vi "Secure WebSocket Client Test with dotNET - Read Timeout.vi"() -> ()   [LabVIEW 2013]
uses:
  dotNET SSL Socket/dotNET WebSocket/Client/SSL Client Options.ctl
  dotNET SSL Socket/dotNET SSL Socket/PFX Certificate.ctl
  dotNET SSL Socket/dotNET WebSocket/Client/dotNET WebSocket Client.lvclass
  <vilib>/MediaMongrels Ltd/WebSockets/WebSockets/WebSocket/WebSocket.lvclass/WebSocket.ctl
  <vilib>/MediaMongrels Ltd/WebSockets/WebSockets/WebSocket/Read Return Headers.vi
  <vilib>/MediaMongrels Ltd/WebSockets/WebSockets/WebSocket Client/WebSocket Client.lvclass
  dotNET SSL Socket/dotNET SSL Client/dotNET SSL Client Socket.lvclass
  dotNET SSL Socket/dotNET TCP Socket/dotNET TCP Socket.lvclass
  dotNET SSL Socket/dotNET SSL Socket/dotNET SSL Socket.lvclass
  NI OpenSSL Socket/SSL_Lib/SSL-Lib/SSL-Lib.lvclass
panel:
  out "x-y":u32
  out "error out 3":errorcluster
  out "Data 3":string
  out "error out 2":errorcluster
  out "error out":errorcluster
  out "Data":string
  out "Return Headers":variant
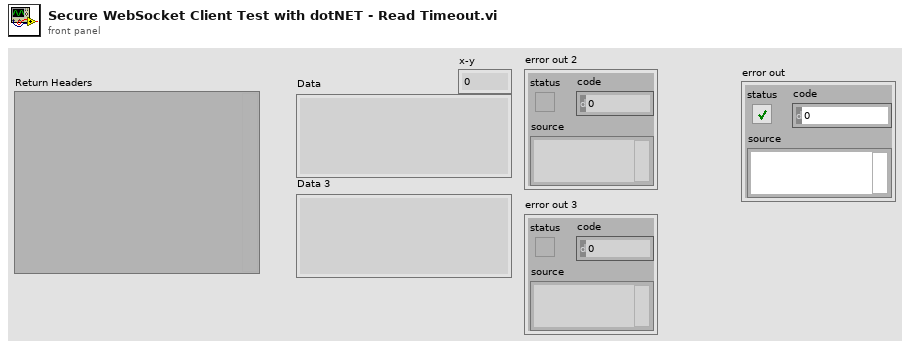
[diagram p1: front panel]
types:
  T1 = typedef "dotNET WebSocket.lvlib/dotNET WebSocket Client.lvclass/SSL Client Options.ctl" = cluster{"Check Revocation":bool, "SSL Protocols":i32[], "Client Certs":T2[]}
  T2 = typedef "dotNET SSL Socket.lvlib/dotNET SSL Socket.lvclass/PFX Certificate.ctl" = cluster{"PFX Certificate":path, "PFX Password":string}
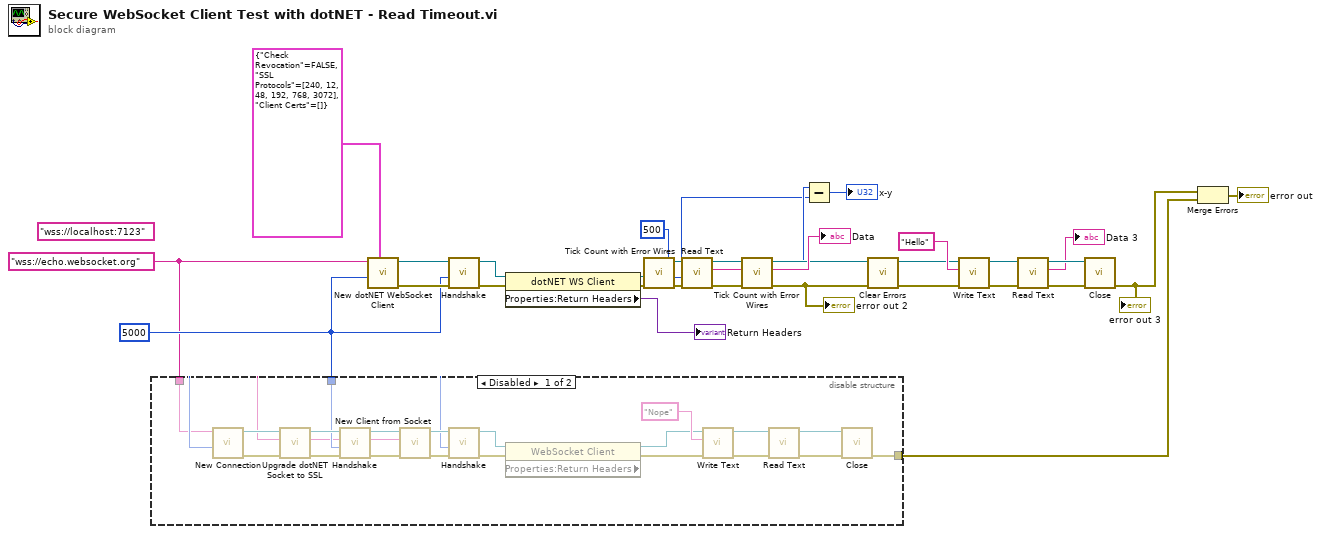
[diagram p0: block diagram]
diagram:
  (unwired) "wss://localhost:7123" ("WebSocket URL")
  w21 = 5000 ("Timeout (5000ms)")
  w19 = "wss://echo.websocket.org" ("WebSocket URL")
  n1 = disable-structure shown="Disabled" {
    disable-tunnel: [w51 _] -> w25
    disable-tunnel: w21 -> [w31 _]
    disable-tunnel: w19 -> [w30 _]
    frame Disabled {
      n2 = call "New Connection.vi"("Timeout (5000ms)"=w31, "Hostname / URL"=w30) -> ("error out"=w32:errorcluster, "dotNET TCP Socket out"=w36:refnum<class "dotNET TCP Socket.lvclass">)  [unwired: 8 in]
      n3 = call "Upgrade dotNET Socket to SSL.vi"("error in (no error)"=w32, "Hostname / URL"=w30, "dotNET TCP Socket in"=w36) -> ("error out"=w33:errorcluster, "dotNET SSL Client Socket out"=w37:refnum<class "dotNET SSL Client Socket.lvclass">)  [unwired: 7 in]
      n4 = call-dynamic "Handshake.vi"("error in (no error)"=w33, "Timeout (5000ms)"=w31, "dotNET SSL Client Socket in"=w37) -> ("error out"=w34:errorcluster, "dotNET SSL Client Socket out"=w35:refnum<class "dotNET SSL Client Socket.lvclass">)  [unwired: 7 in]
      n5 = call <vilib>:"New Client from Socket.vi"("error in (no error)"=w34, "WebSocket URL"=w30, "Socket in"=w35) -> ("error out"=w38:errorcluster, "WebSocket Client out"=w39:refnum<class "WebSocket Client.lvclass">)  [unwired: 7 in]
      n6 = call-dynamic "Handshake.vi"("error in (no error)"=w38, "timeout ms (5000)"=w31, "WebSocket Client in"=w39) -> ("error out"=w40:errorcluster, "WebSocket Client out"=w41:refnum<class "WebSocket Client.lvclass">)  [unwired: 7 in]
      n7 = property class="WebSocket Client"(reference=w41, error in=w40) -> (reference out=w44:refnum<class "WebSocket Client.lvclass">, error out=w43:errorcluster, "Properties:Return Headers"=w42:variant)
      n8 = call-dynamic "Write Text.vi"("error in (no error)"=w43, "String Data"="Nope", "WebSocket in"=w44) -> ("error out"=w46:errorcluster, "WebSocket out"=w47:refnum<class "WebSocket Client.lvclass">)  [unwired: 7 in]
      n9 = call-dynamic "Read Text.vi"("error in (no error)"=w46, "WebSocket in"=w47) -> ("error out"=w49:errorcluster, "Data"=w48:string, "WebSocket out"=w50:refnum<class "WebSocket Client.lvclass">)  [unwired: 7 in]
      n10 = call-dynamic "Close.vi"("error in (no error)"=w49, "WebSocket in"=w50) -> ("error out"=w51:errorcluster)  [unwired: 9 in]
    }
    frame Enabled {
    }
  }
  n11 = call "New dotNET WebSocket Client.vi"("Client SSL Options (wss://)"=T1 {"Check Revocation"=FALSE, "SSL Protocols"=[240, 12, 48, 192, 768, 3072], "Client Certs"=[]} ("SSL Options (for wss://)"), "Timeout (5000ms)"=w21, "WebSocket URL"=w19) -> ("error out"=w23:errorcluster, "dotNET WS Client out"=w22:refnum<class "dotNET WebSocket Client.lvclass">)  [unwired: 7 in]
  n12 = call-dynamic "Handshake.vi"("error in (no error)"=w23, "timeout ms (5000)"=w21, "WebSocket Client in"=w22) -> ("error out"=w29:errorcluster, "WebSocket Client out"=w28:refnum<class "dotNET WebSocket Client.lvclass">)  [unwired: 7 in]
  n13 = property class="dotNET WS Client"(reference=w28, error in=w29) -> (reference out=w15:refnum<class "dotNET WebSocket Client.lvclass">, error out=w16:errorcluster, "Properties:Return Headers"=→"Return Headers":variant)
  n14 = call "Tick Count with Error Wires.vi"("error in (no error)"=w16) -> ("error out"=w4:errorcluster, "millisecond timer value"=w2:u32)  [unwired: 9 in]
  n15 = call-dynamic "Read Text.vi"("error in (no error)"=w4, "timeout ms (5000)"=500, "WebSocket in"=w15) -> ("error out"=w7:errorcluster, "Data"=→"Data":string, "WebSocket out"=w14:refnum<class "dotNET WebSocket Client.lvclass">)  [unwired: 6 in]
  n16 = call "Tick Count with Error Wires.vi"("error in (no error)"=w7) -> ("error out"=w5:errorcluster, "millisecond timer value"=w3:u32)  [unwired: 9 in]
  "error out 2" <- w5
  n17 = Subtract(x=w3, y=w2) -> (x-y=→"x-y":u32)
  n18 = call <vilib>:"Clear Errors.vi"("error in (no error)"=w5) -> ("error out"=w6:errorcluster)  [unwired: 6 in]
  n19 = call-dynamic "Write Text.vi"("error in (no error)"=w6, "String Data"="Hello", "WebSocket in"=w14) -> ("error out"=w13:errorcluster, "WebSocket out"=w11:refnum<class "dotNET WebSocket Client.lvclass">)  [unwired: 7 in]
  n20 = call-dynamic "Read Text.vi"("error in (no error)"=w13, "WebSocket in"=w11) -> ("error out"=w12:errorcluster, "Data"=→"Data 3":string, "WebSocket out"=w10:refnum<class "dotNET WebSocket Client.lvclass">)  [unwired: 7 in]
  n21 = call-dynamic "Close.vi"("error in (no error)"=w12, "WebSocket in"=w10) -> ("error out"=w26:errorcluster)  [unwired: 9 in]
  "error out 3" <- w26
  n22 = Merge Errors(w26, w25) -> (→"error out":errorcluster)
